vi "Append to Array - Null.vi"(0 "JSON Tree in (JSON Array)":variant, 11 "error in (no error)":errorcluster) -> (4 "JSON Tree out (JSON Array)":variant, 15 "error out":errorcluster)   [LabVIEW 2015, in "i3-json.lvlib"]
doc: "Appends a null value to the given array"
uses:
  i3-json.lvlib
  JSON Types/JSON Type.ctl
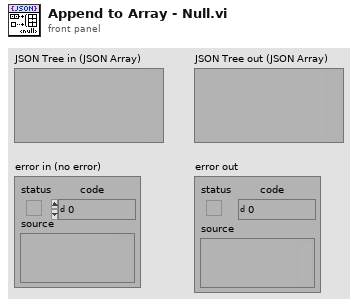
[diagram p1: front panel]
types:
  T1 = typedef "i3-json.lvlib/JSON Type.ctl" = enum8{"JSON Compatible", "JSON Array", "JSON Object", "JSON Null", "Double", "String", "Boolean", "Unknown"}
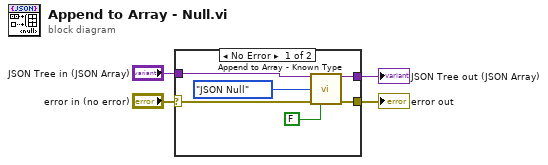
[diagram p0: block diagram]
diagram:
  n1 = case shown="No Error" "error in (no error)" {
    selector: "error in (no error)" -> [w8 w12]
    tunnel: [w9 w12] -> w3
    tunnel: [w10 w11] -> w2
    tunnel: "JSON Tree in (JSON Array)" -> [w7 w11]
    frame No Error {
      n2 = call "Append to Array - Known Type.vi"("JSON Tree in (JSON Array)"=w7, "JSON Type"=JSON_Type."JSON Null", "error in (no error)"=w8, "Add Parameter as JSON Tree?"=FALSE) -> ("JSON Tree out (JSON Array)"=w10:variant, "error out"=w9:errorcluster)  [unwired: 10 in]
    }
    frame Error {
    }
  }
  "error out" <- w3
  "JSON Tree out (JSON Array)" <- w2
